vi "calculate_derived_values.vi"(11 "scan specification":T2) -> (3 "derived values":T1)   [LabVIEW 2010]
uses:
  scan_specification_cluster.ctl
  derived_values_cluster.ctl
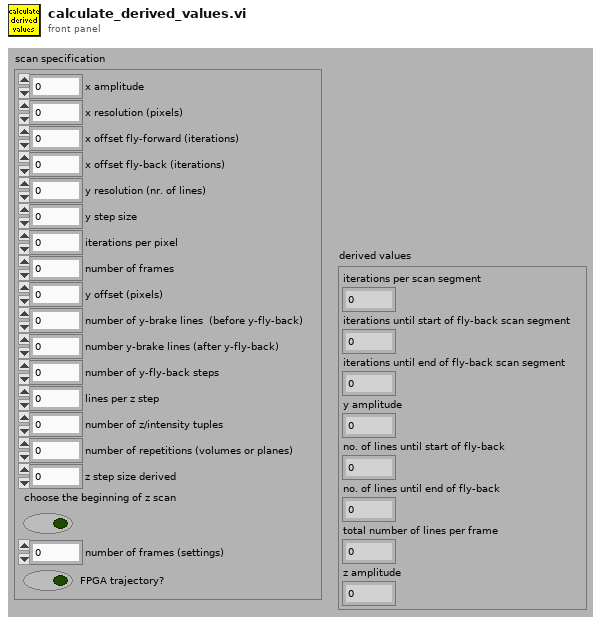
[diagram p1: front panel]
types:
  T1 = typedef "derived_values_cluster.ctl" = cluster{"iterations per scan segment":u16, "iterations until start of fly-back scan segment":u16, "iterations until end of fly-back scan segment":u16, "y amplitude":u16, "no. of lines until start of fly-back":u16, "no. of lines until end of fly-back":u16, "total number of lines per frame ":u16, "z amplitude":u16}
  T2 = typedef "scan_specification_cluster.ctl" = cluster{"x amplitude":u16, "x resolution (pixels)":u16, "x offset fly-forward (iterations)":u16, "x offset fly-back (iterations)":u16, "y resolution (nr. of lines)":u16, "y step size":u16, "iterations per pixel":u16, "number of frames":i32, "y offset (pixels)":u16, "number of y-brake lines  (before y-fly-back)":u16, "number y-brake lines (after y-fly-back)":u16, "number of y-fly-back steps":u16, "lines per z step":u16, "number of z/intensity tuples":u16, "number of repetitions (volumes or planes)":i32, "z step size derived":u16, "choose the beginning of z scan":bool, "number of frames (settings)":i32, "FPGA trajectory?":bool}
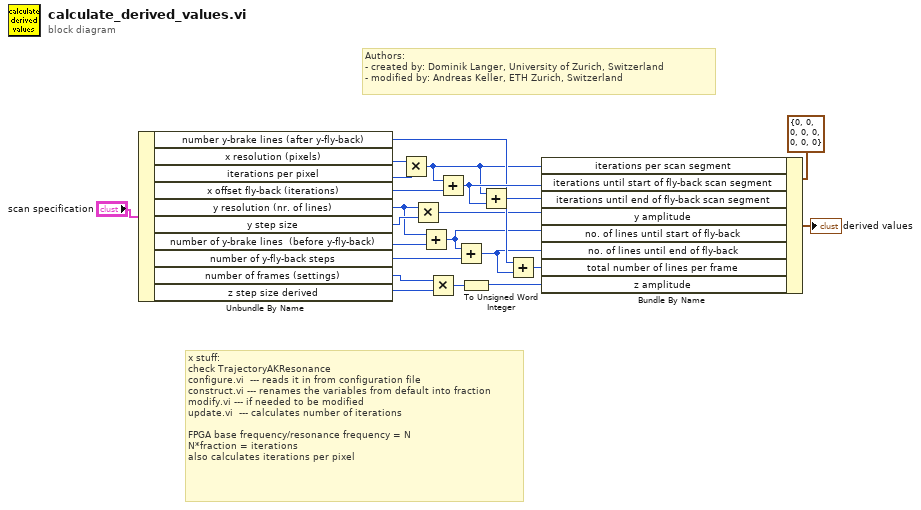
[diagram p0: block diagram]
diagram:
  # "x stuff:\ncheck TrajectoryAKResonance\nconfigure.vi  --- reads it in from configuration file\nconstruct.vi --- renames the variables from default into fraction\nmodify.vi --- if needed to be modified\nupdate.vi  --- calculates number of iterations\n\nFPGA base frequency/resonance frequency = N\nN*fraction = iterations\nalso calculates iterations per pixel"
  # "Authors: \n- created by: Dominik Langer, University of Zurich, Switzerland\n- modified by: Andreas Keller, ETH Zurich, Switzerland"
  n1 = Unbundle By Name("scan specification") -> ("number y-brake lines (after y-fly-back)"=w11:u16, "x resolution (pixels)"=w19:u16, "iterations per pixel"=w18:u16, "x offset fly-back (iterations)"=w17:u16, "y resolution (nr. of lines)"=w13:u16, "y step size"=w14:u16, "number of y-brake lines  (before y-fly-back)"=w12:u16, "number of y-fly-back steps"=w2:u16, "number of frames (settings)"=w4:i32, "z step size derived"=w7:u16)
  n2 = Multiply(x=w19, y=w18) -> (x*y=w9:u16)
  n3 = Multiply(x=w13, y=w14) -> (x*y=w1:u16)
  n4 = Add(x=w13, y=w12) -> (x+y=w3:u16)
  n5 = Multiply(x=w4, y=w7) -> (x*y=w6:i32)
  n6 = Add(x=w9, y=w17) -> (x+y=w16:u16)
  n7 = Add(x=w3, y=w2) -> (x+y=w10:u16)
  n8 = To Unsigned Word Integer(number=w6) -> (unsigned 16bit integer=w5:u16)
  n9 = Add(x=w9, y=w16) -> (x+y=w15:u16)
  n10 = Add(x=w11, y=w10) -> (x+y=w8:u16)
  n11 = Bundle By Name(cluster=T1 {"iterations per scan segment"=0, "iterations until start of fly-back scan segment"=0, "iterations until end of fly-back scan segment"=0, "y amplitude"=0, "no. of lines until start of fly-back"=0, "no. of lines until end of fly-back"=0, "total number of lines per frame "=0, "z amplitude"=0} ("derived values"), "iterations per scan segment"=w9, "iterations until start of fly-back scan segment"=w16, "iterations until end of fly-back scan segment"=w15, "y amplitude"=w1, "no. of lines until start of fly-back"=w3, "no. of lines until end of fly-back"=w10, "total number of lines per frame"=w8, "z amplitude"=w5) -> (→"derived values":T1)
